vi "get current directory.vi"() -> (0 "Current Directory":path)   [LabVIEW 2021]
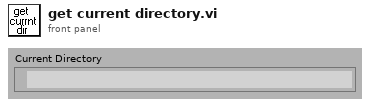
[diagram p1: front panel]
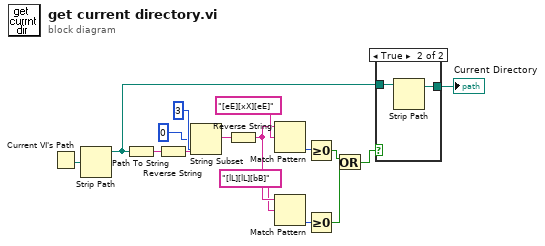
[diagram p0: block diagram]
diagram:
  n1 = Current VI's Path() -> (path=w16:path)
  n2 = Strip Path(path=w16) -> (stripped path=w8:path)  [unwired: 1 out]
  n3 = Path To String(path=w8) -> (string=w15:string)
  n4 = Reverse String(1:w15) -> (0:w14:string)
  n5 = String Subset(string=w14, offset (0)=0, length (rest)=3 ("length")) -> (substring=w11:string)
  n6 = Reverse String(1:w11) -> (0:w6:string)
  n7 = Match Pattern(string=w6, regular expression="[eE][xX][eE]") -> (offset past match=w9:i32)  [unwired: 1 in, 3 out]
  n8 = Match Pattern(string=w6, regular expression="[lL][lL][bB]") -> (offset past match=w3:i32)  [unwired: 1 in, 3 out]
  n9 = Greater Or Equal To 0?(x=w9) -> (x >= 0?=w4:bool)
  n10 = Greater Or Equal To 0?(x=w3) -> (x >= 0?=w2:bool)
  n11 = Or(x=w4, y=w2) -> (x .or. y?=w1:bool)
  n12 = case shown="True" w1 {
    tunnel: w8 -> [w17 w19]
    tunnel: [w17 w18] -> w7
    frame False {
    }
    frame True {
      n13 = Strip Path(path=w19) -> (stripped path=w18:path)  [unwired: 1 out]
    }
  }
  "Current Directory" <- w7
